vi "LVFunction_Imop_Pupil_ApplyShutOfBoundaries.vi"(0 "Pupil in":refnum<class "Pupil.lvclass">, 5 "Pupil OUT":refnum<class "Pupil.lvclass">, 7 "ShutOfBoundaries":u32, 11 "error in (no error)":errorcluster) -> (4 "Pupil out":refnum<class "Pupil.lvclass">, 6 "Pupil OUT 2":refnum<class "Pupil.lvclass">, 15 "error out":errorcluster)   [LabVIEW 2020]
doc: "Applies a \"ShutOfBoundaries\" (Erosion) to a Pupil object.\n\n<B>Pupil_inIn</B> : Pupil object, modified by the operation if Pupil_out = NULL.\n<B>Pupil_inOut</B> : Pupil object, modified by the operation if Pupil_out = NULL.\n<B>shutoff_radius</B> : Radius of the boundary neighbourood where sub-pupils must be shut off.\n<B>Pupil_out</B> : processed Pupil object if not NULL."
uses:
  Pupil.lvclass
  LVClass_Pupil Read Pupil.vi
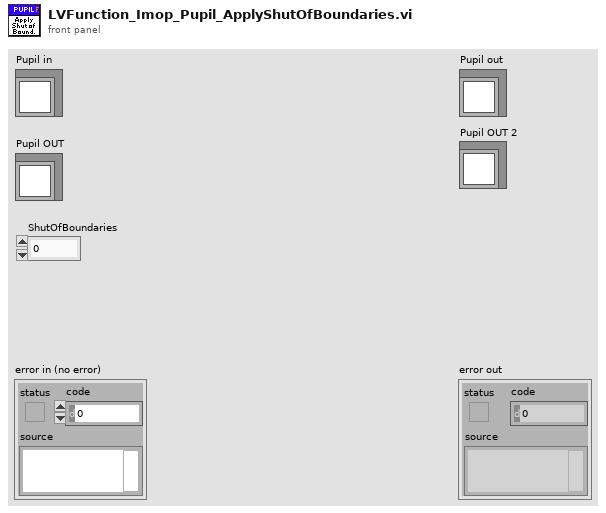
[diagram p1: front panel]
types:
  T1 = typedef "ClassID.ctl" = i64
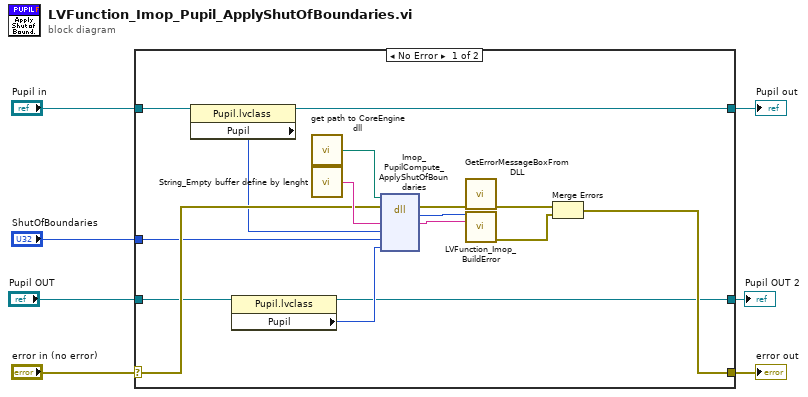
[diagram p0: block diagram]
diagram:
  n1 = case shown="No Error" "error in (no error)" {
    selector: "error in (no error)" -> [w16 w25]
    tunnel: [w15 w25] -> w6
    tunnel: [w9 w24] -> w4
    tunnel: "Pupil in" -> [w10 w24]
    tunnel: "Pupil OUT" -> [w14 _]
    tunnel: [w12 _] -> w2
    tunnel: "ShutOfBoundaries" -> [w11 _]
    frame No Error {
      n2 = property class="Pupil.lvclass"(reference=w10) -> (reference out=w9:refnum<class "Pupil.lvclass">, "Pupil"=w8:T1)  [unwired: 1 in, 1 out]
      n3 = property class="Pupil.lvclass"(reference=w14) -> (reference out=w12:refnum<class "Pupil.lvclass">, "Pupil"=w13:T1)  [unwired: 1 in, 1 out]
      n4 = call "get path to CoreEngine dll.vi"() -> ("path to wavekit library"=w20:path)  [unwired: 14 in, 1 out]
      n5 = call "String_Empty buffer define by lenght.vi"() -> ("Empty buffer"=w23:string)  [unwired: 1 in]
      n6 = dll-call lib="D:/FLE/0.Code/CoreEngine4_Suite/LV2011_interface/DLLs/c_interface_vc100.dll" fn="Imop_PupilCompute_ApplyShutOfBoundaries"(path in=w20, error in=w16, "message"=w23, "Pupil IN"=w8, "ShutOfBoundaries"=w11, "Pupil OUT"=w13) -> (error out=w19:errorcluster, "return type"=w21:u32, "message"=w22:string)  [unwired: 4 in, 1 out]
      n7 = call "GetErrorMessageBoxFromDLL.vi"("error IN"=w19) -> ("error OUT"=w18:errorcluster)  [unwired: 10 in]
      n8 = call "LVFunction_Imop_BuildError.vi"("code"=w21, "String to Prepend to source (\"\")"=w22) -> ("error out"=w17:errorcluster)  [unwired: 13 in]
      n9 = Merge Errors(w18, w17) -> (w15:errorcluster)
    }
    frame Error {
    }
  }
  "error out" <- w6
  "Pupil out" <- w4
  "Pupil OUT 2" <- w2
